vi "timer.vi"   [LabVIEW 2012]
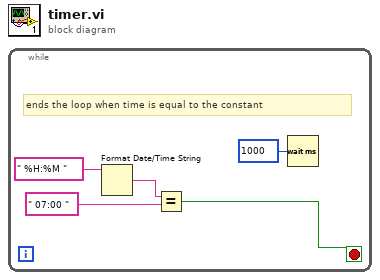
[diagram p0: block diagram]
diagram:
  n1 = while {
    stop <- w1 stop-if-true
    # "ends the loop when time is equal to the constant"
    n2 = Format Date/Time String(time format string (%c)=" %H:%M ") -> (date/time string=w2:string)  [unwired: 2 in]
    n3 = Equal?(x=w2, y=" 07:00 " ("time format string (%c)")) -> (x = y?=w1:bool)
    n4 = Wait (ms)(milliseconds to wait=u32 1000) -> ()  [unwired: 1 out]
  }
